vi "DAQmx Write (Counter 1D Frequency NChan 1Samp).vi"(0 "task/channels in":refnum<k21>, 1 "auto start":bool=TRUE, 7 "data":cluster{"duty cycle":dbl, "frequency":dbl}[](array[cluster]), 9 "timeout":dbl=10.0 format="%0.2f", 11 "error in":errorcluster) -> (4 "task out":refnum<k21>, 10 "number of samples written per channel":u32, 15 "error out":errorcluster)   [LabVIEW 2013]
doc: "Writes a new pulse frequency and duty cycle to each channel in a counter output task that contains one or more channels."
uses:
  nilvaiu.dll
panel:
  # "channel"
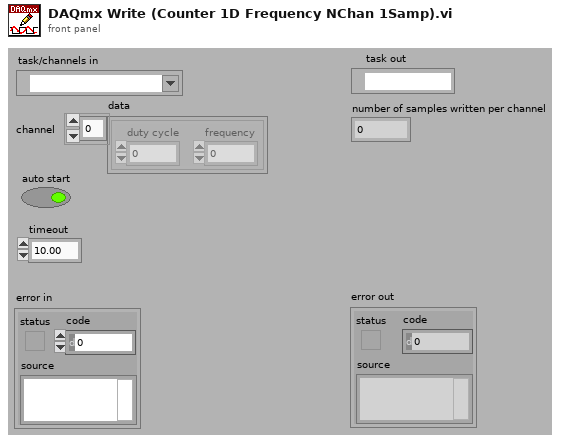
[diagram p1: front panel]
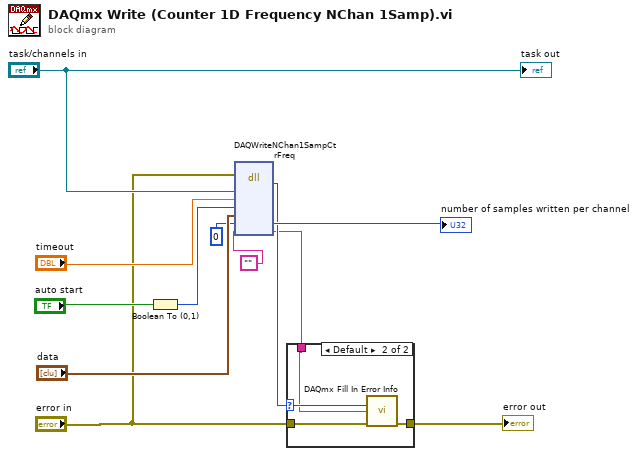
[diagram p0: block diagram]
diagram:
  n1 = Boolean To (0,1)(Boolean="auto start") -> (0, 1=w5:i16)
  n2 = dll-call lib="nilvaiu.*" fn="DAQWriteNChan1SampCtrFreq"(error in="error in", "taskID"="task/channels in", "timeout"="timeout", "autoStart"=w5, "data"="data", "numSamplesWriten"=u32 0, "extendedErrorInfo"="") -> (w6:i32, "numSamplesWriten"=→"number of samples written per channel":u32, "extendedErrorInfo"=w4:string)  [unwired: 4 in, 4 out]
  n3 = case shown="Default" w6 {
    selector: w6 -> [_ w15]
    tunnel: "error in" -> [w13 w17]
    tunnel: [w13 w16] -> w11
    tunnel: w4 -> [_ w14]
    frame 0 {
    }
    frame Default {
      n4 = call "DAQmx Fill In Error Info.vi"("status code"=w15, "extended error info"=w14, "error in"=w17) -> ("error out"=w16:errorcluster)  [unwired: 1 in, 11 out]
    }
  }
  "error out" <- w11
  "task out" <- "task/channels in"
